vi "CoersionDot.vi"() -> ()   [LabVIEW 2019]
panel:
  out "U8":u8
  in  "U16":u16
  out "U16":u16
  in  "U8":u8
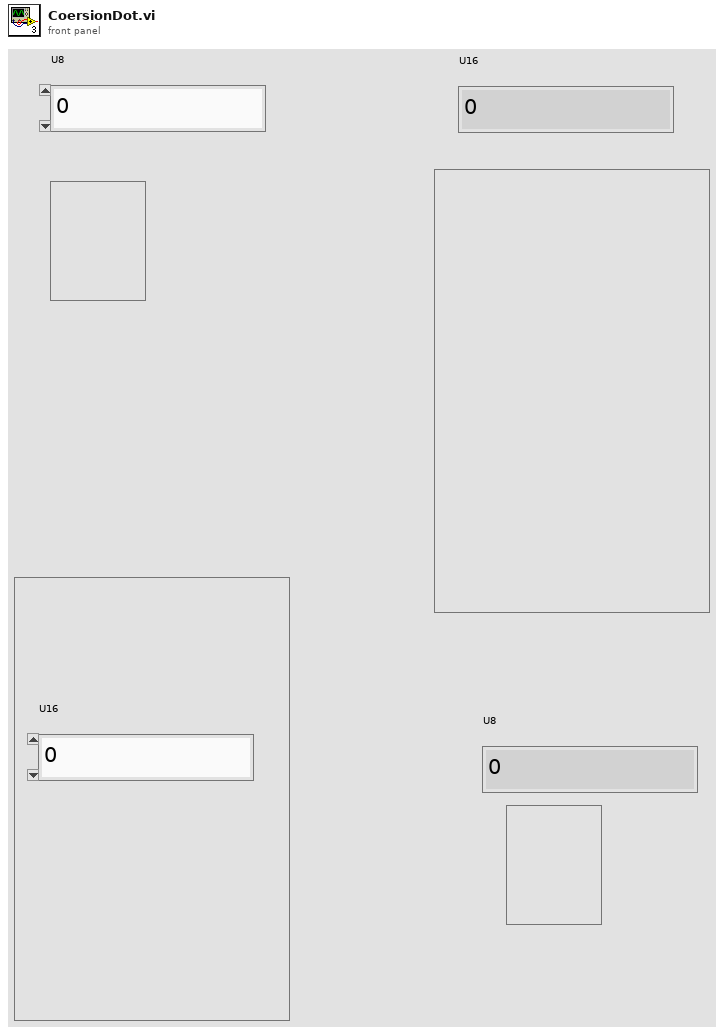
[diagram p1: front panel]
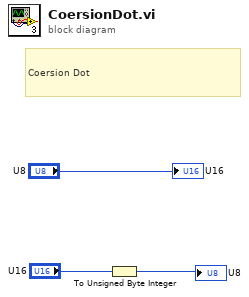
[diagram p0: block diagram]
diagram:
  # "Coersion Dot"
  n1 = To Unsigned Byte Integer(number="U16") -> (unsigned 8bit integer=→"U8":u8)
  "U16" <- "U8"
